vi "Create State.vi"(8 "error in (no error)":errorcluster, 11 "Thread in":refnum<class "Thread.lvclass">) -> (0 "error out":errorcluster, 3 "Thread out":refnum<class "Thread.lvclass">)   [LabVIEW 2019, in "DSF Core.lvlib" / "Thread.lvclass"]
uses:
  Thread.lvclass
  Thread State.ctl
  <vilib>/NI/Memory Manager/Classes/Pointer/Pointer.lvclass
  <vilib>/NI/Memory Manager/Classes/Pointer/Pointer.lvclass/Pointer.ctl
  Thread.lvclass/Thread.ctl
  <vilib>/NI/Memory Manager/Classes/Pointer/Set Address.vi
  <vilib>/NI/Memory Manager/Classes/Pointer/Set Size.vi
  <vilib>/NI/Memory Manager/Classes/Pointer/Set Internal.vi
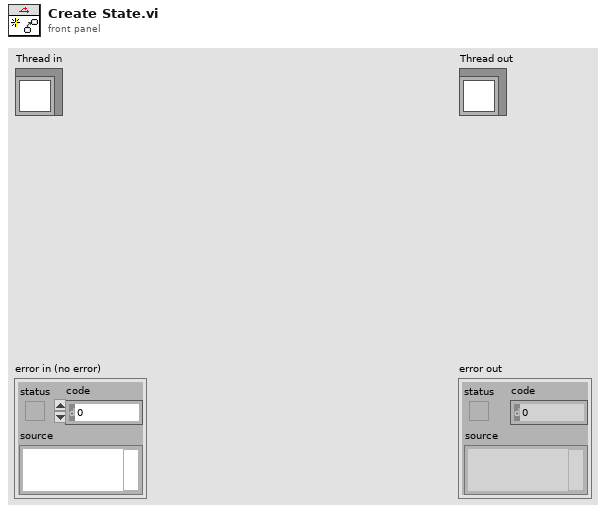
[diagram p1: front panel]
types:
  T1 = typedef "DSF Core.lvlib/Thread.lvclass/Thread State.ctl" = enum8{"Idle", "Running", "Error", "Shut Down"}
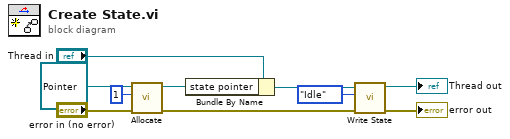
[diagram p0: block diagram]
diagram:
  n1 = call <vilib>:"Allocate.vi"("error in (no error)"="error in (no error)", "size"=u64 1 ("count (1)"), "Pointer type"=refnum<class "Pointer.lvclass"> refnum ("Pointer in")) -> ("error out"=w3:errorcluster, "Pointer out"=w8:refnum<class "Pointer.lvclass">)  [unwired: 7 in]
  n2 = Bundle By Name(cluster="Thread in", "state pointer"=w8) -> (w4:refnum<class "Thread.lvclass">)
  n3 = call "Write State.vi"("error in (no error)"=w3, "state"=Thread_State."Idle", "Thread in"=w4) -> ("error out"=→"error out":errorcluster, "Thread out"=→"Thread out":refnum<class "Thread.lvclass">)  [unwired: 7 in]
